vi "comm options.vi"(8 "error in (no error)":errorcluster, 10 "options string":string, 11 "Comm Handle":u32) -> (0 "error out":errorcluster, 3 "dup Comm Handle":u32)   [LabVIEW 2017, in "lvserial.lvlib"]
doc: "Sets the serial port options. This function is also called inside the CommOpen function and allows the user to specify the major settings together with the serial port name in one string."
uses:
  lvserial.lvlib
  lvserial.dll
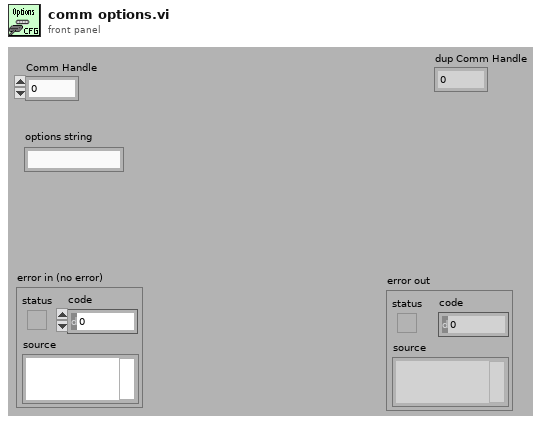
[diagram p1: front panel]
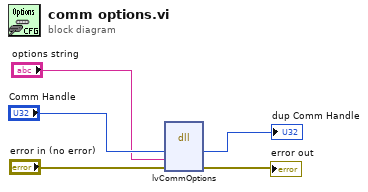
[diagram p0: block diagram]
diagram:
  n1 = dll-call lib="lvserial.dll" fn="lvCommOptions"("hComm"="Comm Handle", "shOptions"="options string", "error in (no error)"="error in (no error)") -> ("hComm"=→"dup Comm Handle":u32, "error in (no error)"=→"error out":errorcluster)  [unwired: 4 in, 3 out]
